vi "串口配置.vi"(9 "PORT":string="1001", 10 "IP":string="127.0.0.1", 11 "请选择串口:":refnum<visa-resource-name>) -> (0 "PORT 2":string="1001", 1 "IP 2":string="127.0.0.1", 2 "确认 2":bool, 3 "VISA资源名称 2":refnum<visa-resource-name>)   [LabVIEW 2016, in "CODCr库.lvlib"]
panel:
  in  "取消":bool
  in  "确认":bool
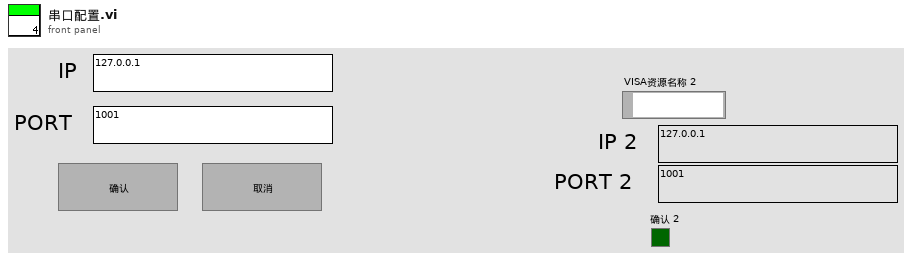
[diagram p1: front panel]
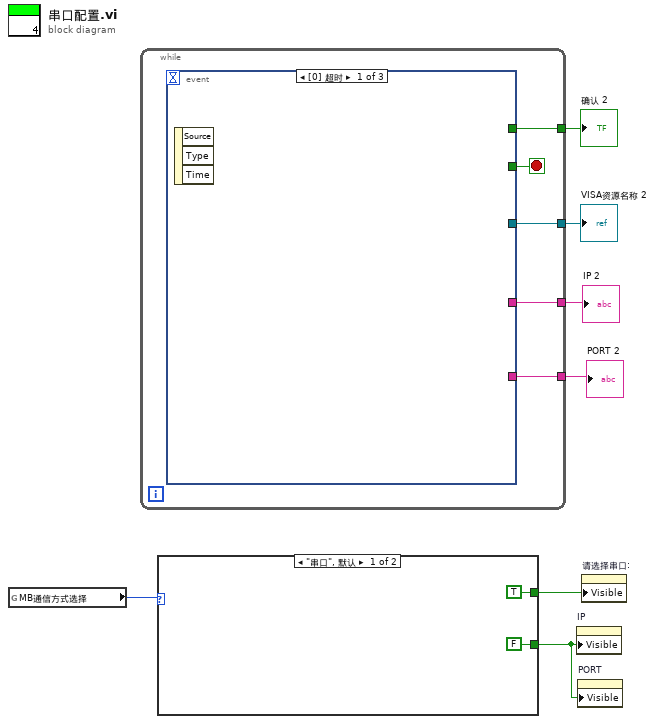
[diagram p0: block diagram]
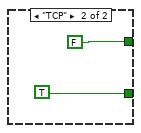
[diagram p2: hidden frame]
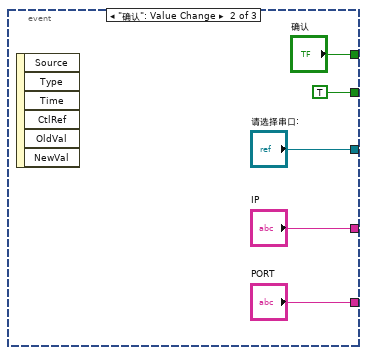
[diagram p3: hidden frame]
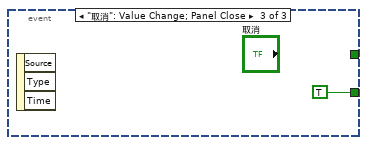
[diagram p4: hidden frame]
diagram:
  n1 = global read "CODcr全局变量.vi" "MB通信方式选择"() -> (w5:enum16{"串口", "TCP"})
  n2 = while {
    tunnel: [w12] -> w7
    tunnel: [w10] -> w6
    tunnel: [w9] -> w4
    tunnel: [w8] -> w3
    stop <- w11 stop-if-true
    n3 = event shown="[0] 超时" {
      selector: _ -> [_ _ _]
      dyn-events: _ -> [_ _ _]
      timeout: _ -> [_ _ _]
      tunnel: [_ "请选择串口:" _] -> w12
      tunnel: [_ TRUE TRUE] -> w11
      tunnel: [_ "确认" _] -> w10
      tunnel: [_ "IP" _] -> w9
      tunnel: [_ "PORT" _] -> w8
      event Timeout {
        n4 = event-data() -> ()  [unwired: 1 in, 3 out]
      }
      event "确认": Value Change {
        n5 = event-data() -> ()  [unwired: 1 in, 6 out]
      }
      event "取消": Value Change; Panel Close {
        n6 = event-data() -> ()  [unwired: 1 in, 3 out]
      }
    }
  }
  "VISA资源名称 2" <- w7
  "确认 2" <- w6
  "IP 2" <- w4
  "PORT 2" <- w3
  n7 = case shown="\"串口\", 默认" w5 {
    tunnel: [FALSE ("可见") TRUE ("可见")] -> w2
    tunnel: [TRUE ("可见") FALSE ("可见")] -> w1
    frame "串口", Default {
    }
    frame "TCP" {
    }
  }
  n8 = property on="IP" class="Str"("Visible"=w2) -> ()  [unwired: 2 in, 2 out]
  n9 = property on="PORT" class="Str"("Visible"=w2) -> ()  [unwired: 2 in, 2 out]
  n10 = property on="请选择串口:" class="VISAName"("Visible"=w1) -> ()  [unwired: 2 in, 2 out]
